vi "Calc_Stats(Global).vi"(7 "No of SubSets":i32, 10 "Local Vars":sgl[](array[numeric]), 11 "Local Means":sgl[](array[numeric])) -> (2 "Global STD":sgl, 3 "Global Mean":sgl)   [LabVIEW 2024]
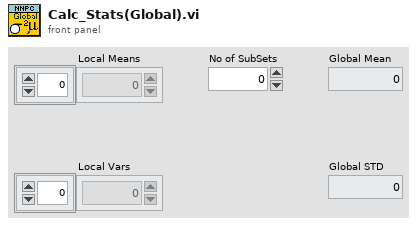
[diagram p1: front panel]
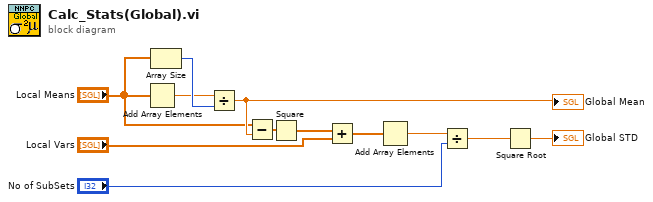
[diagram p0: block diagram]
diagram:
  n1 = Add Array Elements(numeric array="Local Means") -> (sum=w1:sgl)
  n2 = Array Size(array="Local Means") -> (size(s)=w2:i32)
  n3 = Divide(x=w1, y=w2) -> (x/y=w12:sgl)
  "Global Mean" <- w12
  n4 = Subtract(x="Local Means", y=w12) -> (x-y=w4:sgl[])
  n5 = Square(x=w4) -> (x^2=w5:sgl[])
  n6 = Add(x=w5, y="Local Vars") -> (x+y=w8:sgl[])
  n7 = Add Array Elements(numeric array=w8) -> (sum=w7:sgl)
  n8 = Divide(x=w7, y="No of SubSets") -> (x/y=w9:sgl)
  n9 = Square Root(x=w9) -> (sqrt(x)=→"Global STD":sgl)
